vi "Seconds to H M S string.vi"(1 "Numeric":dbl) -> (0 "String":string)   [LabVIEW 2012, in "Strings Lib.lvlib"]
uses:
  Strings Lib.lvlib
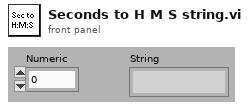
[diagram p1: front panel]
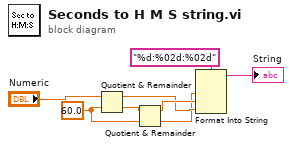
[diagram p0: block diagram]
diagram:
  w6 = 60.0 ("y")
  n1 = Quotient & Remainder(x="Numeric", y=w6) -> (x-y*floor(x/y)=w2:dbl, floor(x/y)=w4:dbl)
  n2 = Quotient & Remainder(x=w4, y=w6) -> (x-y*floor(x/y)=w3:dbl, floor(x/y)=w1:dbl)
  n3 = Format Into String(format string="%d:%02d:%02d", w1, w3, w2) -> (resulting string=→"String":string)  [unwired: 2 in, 1 out]
